vi "setNSteps.vi"(0 "connection ID":i32, 1 "axis":i32, 2 "backward":bool, 3 "step":i32, 5 "error in":errorcluster) -> (14 "connection ID":i32, 15 "axis_out":i32, 19 "error out":errorcluster)   [LabVIEW 2016]
doc: "This function triggers n steps on the selected axis in desired direction."
panel:
  out "params_cluster":cluster{"axis":i32, "backward":bool, "step":i32}
  in  "Params_cluster":T1
  in  "results_cluster":cluster{"errNo":i32}
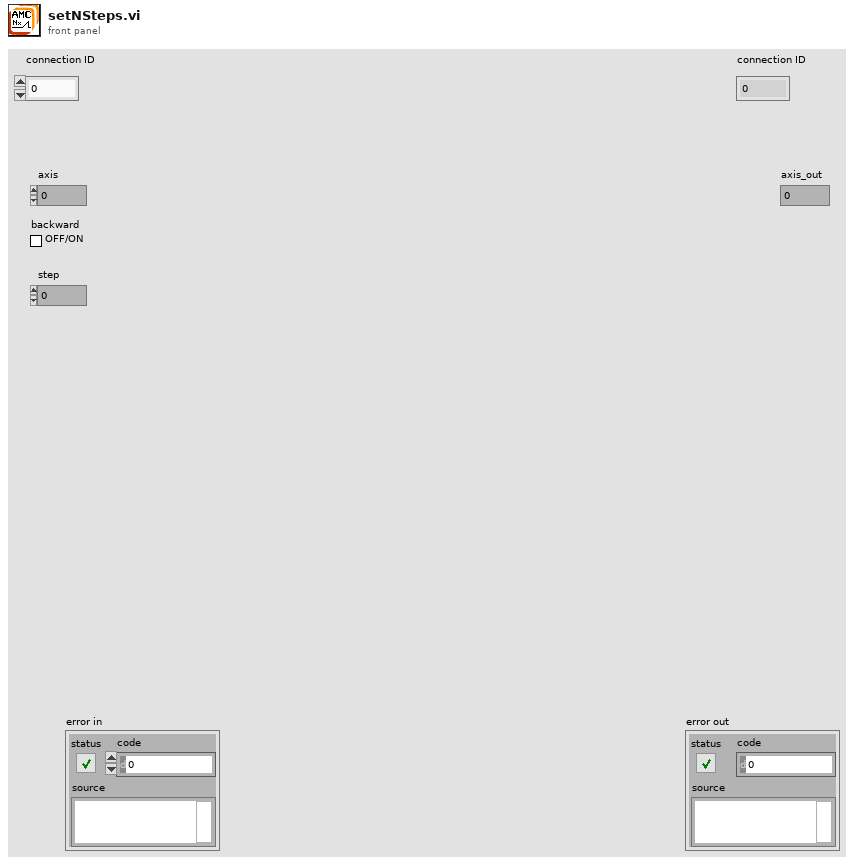
[diagram p1: front panel]
types:
  T1 = cluster{"integer":i32, "boolean":bool, "integer":i32}
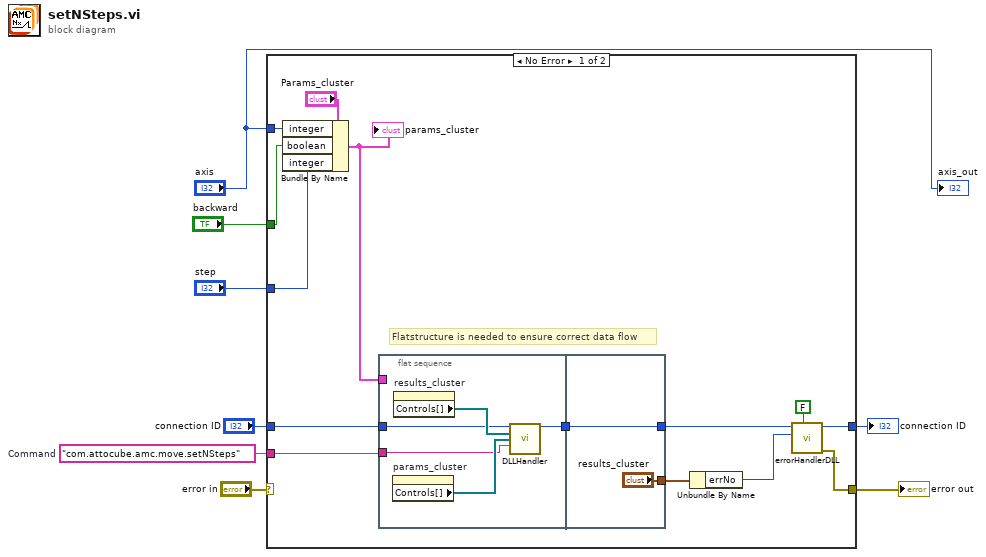
[diagram p0: block diagram]
diagram:
  w6 = "com.attocube.amc.move.setNSteps"  # Command
  n1 = case shown="No Error" "error in" {
    selector: "error in" -> [_ w31]
    tunnel: [w21 w31] -> w8
    tunnel: w6 -> [w16 _]
    tunnel: [w15 w30] -> w5
    tunnel: "connection ID" -> [w14 w30]
    tunnel: "axis" -> [w11 _]
    tunnel: "backward" -> [w10 _]
    tunnel: "step" -> [w9 _]
    frame No Error {
      # "Flatstructure is needed to ensure correct data flow"
      n2 = Bundle By Name(cluster="Params_cluster", "integer"=w11, "boolean"=w10, "integer"=w9) -> (w12:T1)
      "params_cluster" <- w12
      n3 = flat-sequence {
        tunnel: [w27] -> w18
        tunnel: w16 -> [w24]
        tunnel: w14 -> [w23]
        tunnel: w12 -> [_]
        tunnel: ["results_cluster"] -> w19
        tunnel: [w29] -> w20
        tunnel: w18 -> [w29]
        frame #0 {
          n4 = property on="params_cluster" class="Clust (strict)"() -> ("Controls[]"=w25:refnum<vi>[])  [unwired: 2 in, 2 out]
          n5 = property on="results_cluster" class="Clust (strict)"() -> ("Controls[]"=w26:refnum<vi>[])  [unwired: 2 in, 2 out]
          n6 = call "DLLHandler.vi"("connection ID"=w23, "results_cluster"=w26, "params_cluster"=w25, "method"=w24) -> ("connection ID out"=w27:i32)  [unwired: 10 in, 1 out]
        }
        frame #1 {
        }
      }
      n7 = Unbundle By Name(w19) -> ("errNo"=w13:i32)
      n8 = call "errorHandlerDLL.vi"("show popup"=FALSE, "error number"=w13, "connection ID"=w20) -> ("error out"=w21:errorcluster, "connection ID"=w15:i32)  [unwired: 7 in]
    }
    frame Error {
    }
  }
  "error out" <- w8
  "connection ID" <- w5
  "axis_out" <- "axis"
